vi "Format Problems.vi"(8 "error in (no error)":errorcluster, 10 "Problems":string[](array[string])) -> (0 "error out":errorcluster)   [LabVIEW 2020, in "GPackTools.lvlib" / "GPackCLI.lvclass"]
uses:
  GPackCLI.lvclass
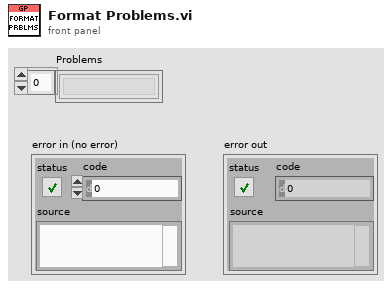
[diagram p1: front panel]
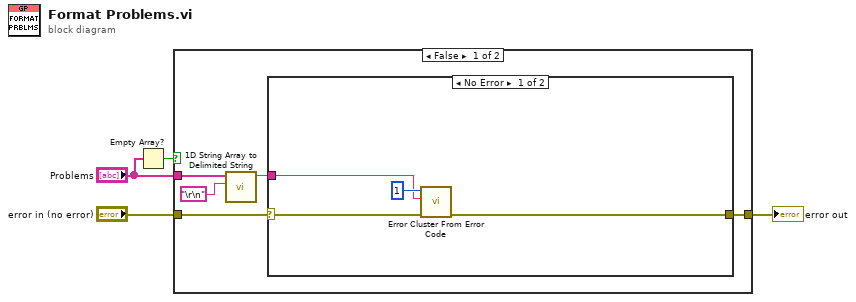
[diagram p0: block diagram]
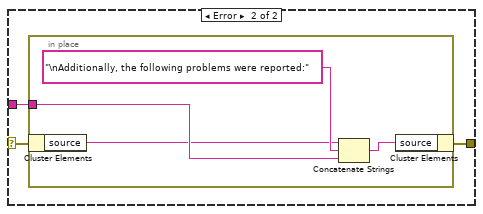
[diagram p2: hidden frame]
diagram:
  n1 = Empty Array?(array="Problems") -> (empty?=w1:bool)
  n2 = case shown="False" w1 {
    tunnel: "error in (no error)" -> [w8 w21]
    tunnel: [w6 w21] -> w3
    tunnel: "Problems" -> [w5 _]
    frame False {
      n3 = call <vilib>:"1D String Array to Delimited String.vi"("delimiter"="\r\n", "string array"=w5) -> ("delimited string"=w7:string)  [unwired: 9 in]
      n4 = case shown="No Error" w8 {
        selector: w8 -> [w13 w16]
        tunnel: w7 -> [w11 w15]
        tunnel: [w10 w14] -> w6
        frame No Error {
          n5 = call <vilib>:"Error Cluster From Error Code.vi"("error in (no error)"=w13, "error message (\"\")"=w11, "error code (0)"=1) -> ("error out"=w10:errorcluster)  [unwired: 6 in]
        }
        frame Error {
          n6 = in-place {
            in-place-border: w15 -> [w19]
            n7 = in-place-cluster #1(w16) -> ("source"=w18:string)
            n8 = Concatenate Strings(w18, "\nAdditionally, the following problems were reported:" ("string"), w19) -> (w17:string)
            n9 = in-place-cluster #1("source"=w17) -> (w14:errorcluster)
          }
        }
      }
    }
    frame True {
    }
  }
  "error out" <- w3
